vi "7-CleanFP2ndMode.vi"   [LabVIEW 2015, in "TestVIs.lvlib"]
uses:
  TestVIs.lvlib
  <vilib>/Utility/miscctls.llb/LVRectTypeDef.ctl
  <vilib>/Utility/traverseref.llb/TRef TravTarget.ctl
  <vilib>/Utility/VariantDataType/Type.ctl
  <vilib>/Utility/VariantDataType/VariantType.lvlib
types:
  T1 = enum32{"Top Edges", "Vertical Centers", "Bottom Edges", "Left Edges", "Horizontal Centers", "Right Edges"}
  T2 = enum32{"Top Edges", "Vertical Centers", "Bottom Edges", "Vertical Gap", "Vertical Compress", "Left Edges", "Horizontal Centers", "Right Edges", "Horizontal Gap", "Horizontal Compress"}
  T3 = typedef "TRef TravTarget.ctl" = enum16{"FP", "BD", "Other"}
  T4 = typedef "LVRectTypeDef.ctl" = cluster{"Left":i16, "Top":i16, "Right":i16, "Bottom":i16}
  T5 = enum16{"Invalid Wire Rule", "Required", "Recommended", "Optional", "Dynamic Dispatch"}
  T6 = enum16{"Invalid Wire Rule", "Required", "Recommended", "Optional", "Dynamic Dispatch"}[]
  T7 = typedef "VariantType.lvlib/Type.ctl" = enum8{"Invalid Type", "Void", "I8", "I16", "I32", "I64", "U8", "U16", "U32", "U64", "Single Float", "Double Float", "Extended Float", "Single Complex", "Double Complex", "Extended Complex", "Enum U8", "Enum U16", "Enum U32", "Enum U64", "Single Float With Unit", "Double Float With Unit", "Extended Float With Unit", "Single Complex with Unit", "Double Complex with Unit", "Extended Complex with Unit", "Boolean", "String", "Path", "Picture", "Tag", "Array", "Cluster", "Variant", "LV Variant", "Waveform", "Timestamp", "Digital Waveform", "Digital Data", "ExpressData", "Refnum", "External Data", "VI", "Poly VI", "LabVIEW Class Instance", "Fixed Point"}
  T8 = cluster{refnum<vi>, "MasterRect":T4, "Type Enum":T7}
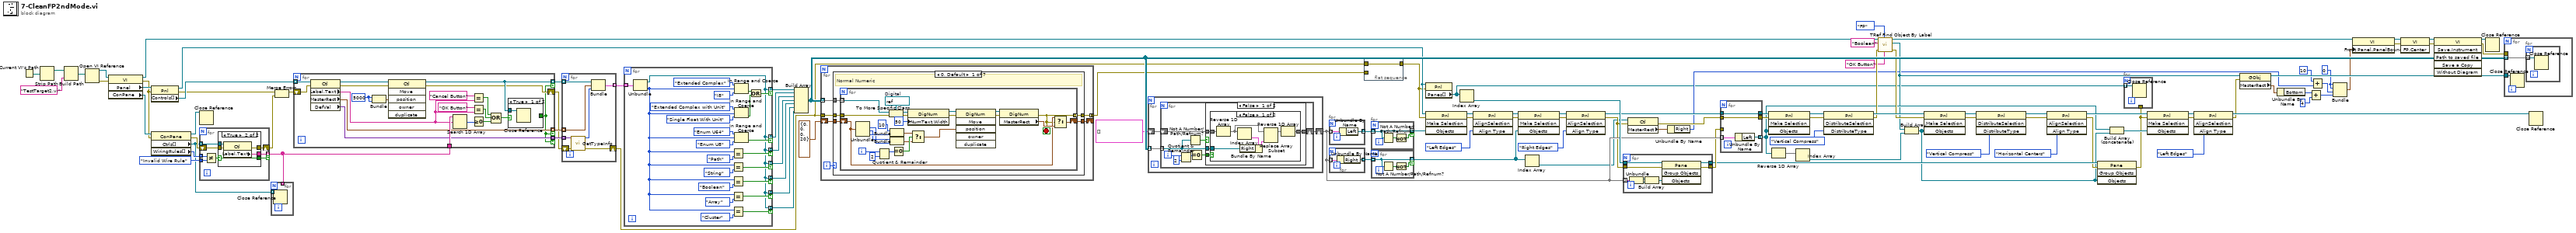
[diagram p0: block diagram]
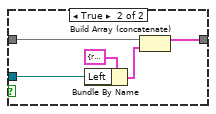
[diagram p2: hidden frame]
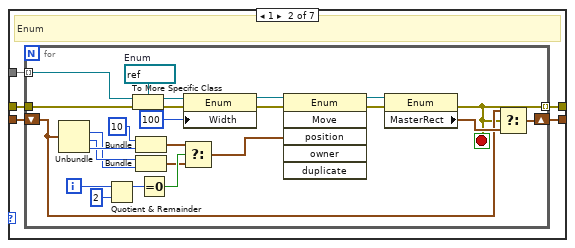
[diagram p4: hidden frame]
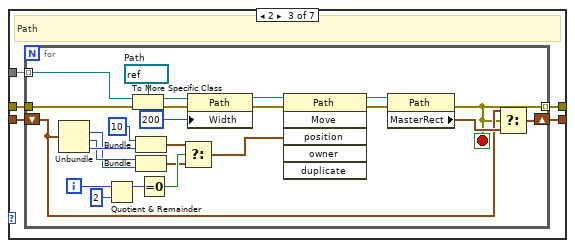
[diagram p5: hidden frame]
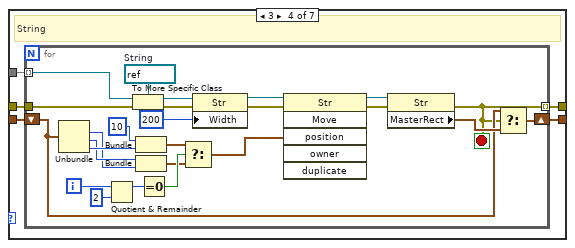
[diagram p6: hidden frame]
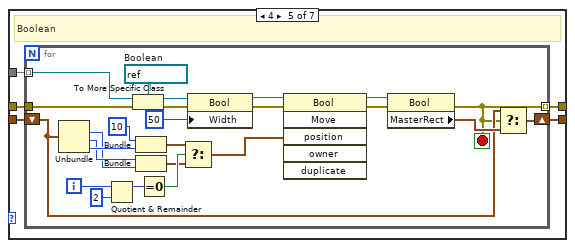
[diagram p7: hidden frame]
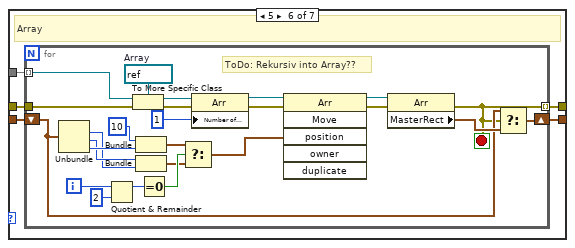
[diagram p8: hidden frame]
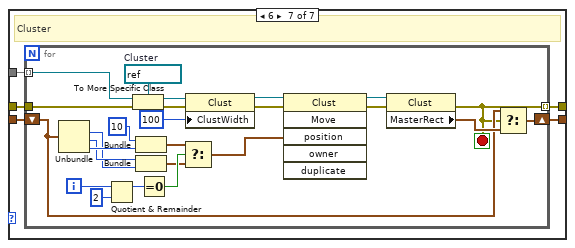
[diagram p9: hidden frame]
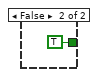
[diagram p10: hidden frame]
diagram:
  w19 = i16 0 ("y")
  n1 = Current VI's Path() -> (path=w106:path)
  n2 = Strip Path(path=w106) -> (stripped path=w109:path)  [unwired: 1 out]
  n3 = Build Path(base path=w109, name or relative path="TestTarget2.vi") -> (appended path=w107:path)
  n4 = Open VI Reference(vi path=w107) -> (vi reference=w93:refnum<vi>, error out=w92:errorcluster)  [unwired: 5 in]
  n5 = property class="VI"(reference=w93, error in=w92) -> (reference out=w52:refnum<vi>, error out=w103:errorcluster, "Panel"=w105:refnum<vi>, "ConPane"=w104:refnum<vi>)
  n6 = property class="Pnl"(reference=w105, error in=w103) -> (reference out=w64:refnum<vi>, error out=w100:errorcluster, "Controls[]"=w101:refnum<vi>[])
  n7 = property class="ConPane"(reference=w104, error in=w103) -> (reference out=w91:refnum<vi>, error out=w102:errorcluster, "Ctrls[]"=w8:refnum<vi>[], "WiringRules[]"=w89:T6)
  n8 = Close Reference(reference=w91) -> ()  [unwired: 1 in, 1 out]
  n9 = for {
    tunnel: w8 -> [w117] mode=indexing
    shift-right: [w115] -> w98
    shift-left: w102 -> [w116]
    tunnel: [w114] -> w7 mode=indexing if=w110
    tunnel: w89 -> [w112] mode=indexing
    tunnel: T5."Invalid Wire Rule" ("Wire Rule") -> [w111]
    n10 = Not Equal?(x=w112, y=w111) -> (x != y?=w113:bool)
    n11 = case shown="True" w113 {
      selector: w113 -> [w118 w120]
      tunnel: w117 -> [_ w124]
      tunnel: w116 -> [w119 w123]
      tunnel: [w119 w122] -> w115
      tunnel: [_ w121] -> w114
      tunnel: [w118 w120] -> w110
      frame False {
      }
      frame True {
        n12 = property class="Ctl"(reference=w124, error in=w123) -> (error out=w122:errorcluster, "Label.Text"=w121:string)  [unwired: 1 out]
      }
    }
  }
  n13 = for {
    tunnel: w8 -> [w125] mode=indexing
    tunnel: w7 -> [_] mode=indexing
    n14 = Close Reference(reference=w125) -> ()  [unwired: 1 in, 1 out]
  }
  n15 = Merge Errors(w100, w98) -> (w99:errorcluster)
  n16 = for {
    tunnel: w101 -> [w145] mode=indexing
    shift-right: [w137] -> w94
    shift-left: w99 -> [w144]
    tunnel: w7 -> [w143]
    tunnel: [w138] -> w95 mode=indexing if=w134
    tunnel: [w136] -> w96 mode=indexing if=w134
    tunnel: [w135] -> w97 mode=indexing if=w134
    w142 = i16 5000 ("x")
    n17 = property class="Ctl"(reference=w145, error in=w144) -> (reference out=w139:refnum<vi>, error out=w140:errorcluster, "Label.Text"=w132:string, "MasterRect"=w136:T4, "DefVal"=w135:variant)
    n18 = Bundle("x"=w142, "x"=w142) -> (w141:cluster{"x":i16, "x":i16})  [unwired: 1 in]
    n19 = invoke class="Ctl" method="Move"(reference=w139, error in=w140, "position"=w141) -> (reference out=w138:refnum<vi>, error out=w137:errorcluster)  [unwired: 3 in, 4 out]
    n20 = Search 1D Array(1D array=w143, element=w132) -> (index of element=w133:i32)  [unwired: 1 in]
    n21 = Equal?(x="Cancel Button", y=w132) -> (x = y?=w131:bool)
    n22 = Equal?(x="OK Button", y=w132) -> (x = y?=w130:bool)
    n23 = Greater Or Equal To 0?(x=w133) -> (x >= 0?=w129:bool)
    n24 = Compound Arithmetic op=OR(w131, w130, w129) -> (w128:bool)
    n25 = case shown="True" w128 {
      tunnel: w138 -> [w146 _]
      tunnel: [_ TRUE] -> w134
      frame True {
        n26 = Close Reference(reference=w146) -> ()  [unwired: 1 in, 1 out]
      }
      frame False {
      }
    }
  }
  n27 = for {
    tunnel: w97 -> [w154] mode=indexing
    tunnel: w96 -> [w152] mode=indexing
    tunnel: w95 -> [w153] mode=indexing
    tunnel: [w151] -> w90 mode=indexing
    shift-right: [w149] -> w66
    shift-left: w94 -> [w150]
    n28 = call <vilib>:"GetTypeInfo.vi"("error in (no error)"=w150, "Variant"=w154) -> ("error out"=w149:errorcluster, "Type Enum"=w148:T7)  [unwired: 5 in, 3 out]
    n29 = Bundle(w153, "MasterRect"=w152, "Type Enum"=w148) -> (w151:T8)  [unwired: 1 in]
  }
  n30 = for {
    tunnel: w90 -> [w157] mode=indexing
    tunnel: [w155] -> w87 mode=indexing if=w171
    tunnel: [w155] -> w86 mode=indexing if=w168
    tunnel: [w155] -> w85 mode=indexing if=w158
    tunnel: [w155] -> w82 mode=indexing if=w166
    tunnel: [w155] -> w81 mode=indexing if=w163
    tunnel: [w155] -> w80 mode=indexing if=w162
    tunnel: [w155] -> w83 mode=indexing if=w156
    n31 = Unbundle(w157) -> (w155:refnum<vi>, "Type Enum"=w159:T7)  [unwired: 1 out]
    n32 = Equal?(x=w159, y=Type."Path" ("Type Enum")) -> (x = y?=w158:bool)
    n33 = Equal?(x=w159, y=Type."String" ("Type Enum")) -> (x = y?=w156:bool)
    n34 = Equal?(x=w159, y=Type."Boolean" ("Type Enum")) -> (x = y?=w166:bool)
    n35 = Equal?(x=w159, y=Type."Array" ("Type Enum")) -> (x = y?=w163:bool)
    n36 = Equal?(x=w159, y=Type."Cluster" ("Type Enum")) -> (x = y?=w162:bool)
    n37 = In Range and Coerce(upper limit=Type."Extended Complex" ("Type Enum"), x=w159, lower limit=Type."I8" ("Type Enum")) -> (In Range?=w173:bool)  [unwired: 1 out]
    n38 = In Range and Coerce(upper limit=Type."Extended Complex with Unit" ("Type Enum"), x=w159, lower limit=Type."Single Float With Unit" ("Type Enum")) -> (In Range?=w172:bool)  [unwired: 1 out]
    n39 = In Range and Coerce(upper limit=Type."Enum U64" ("Type Enum"), x=w159, lower limit=Type."Enum U8" ("Type Enum")) -> (In Range?=w168:bool)  [unwired: 1 out]
    n40 = Or(x=w173, y=w172) -> (x .or. y?=w171:bool)
  }
  n41 = Build Array(w87, w86, w85, w83, w82, w81, w80) -> (w79:refnum<vi>[][])
  n42 = for {
    tunnel: w79 -> [w182] mode=indexing
    shift-right: [w179] -> _
    shift-left: T4 {"Left"=0, "Top"=0, "Right"=0, "Bottom"=20} ("MasterRect") -> [w180]
    tunnel: w66 -> [w183]
    tunnel: [w178] -> w65 mode=concatenating
    i -> [w181]
    n43 = case shown="0, Default" w181 {
      tunnel: w182 -> [w188 w218 w248 w278 w308 w338 w368]
      tunnel: [w187 w217 w247 w277 w307 w337 w367] -> w178
      tunnel: [w186 w216 w246 w276 w306 w336 w366] -> w179
      tunnel: w183 -> [w185 w215 w245 w275 w305 w335 w365]
      tunnel: w180 -> [w184 w214 w244 w274 w304 w334 w364]
      frame 0, Default {
        # "Normal Numeric"
        n44 = for {
          tunnel: w188 -> [w193] mode=indexing
          shift-right: [w192] -> w186
          shift-left: w184 -> [w190]
          tunnel: w185 -> [w212]
          tunnel: [w189] -> w187 mode=indexing
          i -> [w213]
          stop <- w189 stop-if-true
          w194 = refnum<vi> refnum  # Digital
          n45 = Unbundle(w190) -> ("Top"=w195:i16, "Right"=w196:i16, "Bottom"=w197:i16)  [unwired: 1 out]
          n46 = Quotient & Remainder(x=w213, y=2) -> (x-y*floor(x/y)=w203:i32)  [unwired: 1 out]
          n47 = To More Specific Class(target class=w194, reference=w193, error in=w212) -> (specific class reference=w210:refnum<vi>, error out=w209:errorcluster)
          n48 = Bundle("Top"=i16 10, "Bottom"=w197) -> (w200:cluster{"Top":i16, "Bottom":i16})  [unwired: 1 in]
          n49 = Bundle("Right"=w196, "Top"=w195) -> (w199:cluster{"Right":i16, "Top":i16})  [unwired: 1 in]
          n50 = Equal To 0?(x=w203) -> (x = 0?=w202:bool)
          n51 = property class="DigNum"(reference=w210, error in=w209, "NumText.Width"=u32 50 ("Numeric Text.Size:Width")) -> (reference out=w208:refnum<vi>, error out=w207:errorcluster)
          n52 = Select(t=w200, s=w202, f=w199) -> (s? t:f=w201:cluster{"Right":i16, "Top":i16})
          n53 = invoke class="DigNum" method="Move"(reference=w208, error in=w207, "position"=w201) -> (reference out=w205:refnum<vi>, error out=w204:errorcluster)  [unwired: 3 in, 4 out]
          n54 = property class="DigNum"(reference=w205, error in=w204) -> (error out=w189:errorcluster, "MasterRect"=w191:T4)  [unwired: 1 out]
          n55 = Select(t=w190, s=w189, f=w191) -> (s? t:f=w192:T4)
        }
      }
      frame 1 {
        # "Enum"
        n56 = for {
          tunnel: w218 -> [w223] mode=indexing
          shift-right: [w222] -> w216
          shift-left: w214 -> [w220]
          tunnel: w215 -> [w242]
          tunnel: [w219] -> w217 mode=indexing
          i -> [w243]
          stop <- w219 stop-if-true
          w224 = refnum<vi> refnum  # Enum
          n57 = Unbundle(w220) -> ("Top"=w225:i16, "Right"=w226:i16, "Bottom"=w227:i16)  [unwired: 1 out]
          n58 = Quotient & Remainder(x=w243, y=2) -> (x-y*floor(x/y)=w233:i32)  [unwired: 1 out]
          n59 = To More Specific Class(target class=w224, reference=w223, error in=w242) -> (specific class reference=w240:refnum<vi>, error out=w239:errorcluster)
          n60 = Bundle("Top"=i16 10, "Bottom"=w227) -> (w230:cluster{"Top":i16, "Bottom":i16})  [unwired: 1 in]
          n61 = Bundle("Right"=w226, "Top"=w225) -> (w229:cluster{"Right":i16, "Top":i16})  [unwired: 1 in]
          n62 = Equal To 0?(x=w233) -> (x = 0?=w232:bool)
          n63 = Select(t=w230, s=w232, f=w229) -> (s? t:f=w231:cluster{"Right":i16, "Top":i16})
          n64 = property class="Enum"(reference=w240, error in=w239, "Width"=u32 100 ("Numeric Text.Size:Width")) -> (reference out=w238:refnum<vi>, error out=w237:errorcluster)
          n65 = invoke class="Enum" method="Move"(reference=w238, error in=w237, "position"=w231) -> (reference out=w235:refnum<vi>, error out=w234:errorcluster)  [unwired: 3 in, 4 out]
          n66 = property class="Enum"(reference=w235, error in=w234) -> (error out=w219:errorcluster, "MasterRect"=w221:T4)  [unwired: 1 out]
          n67 = Select(t=w220, s=w219, f=w221) -> (s? t:f=w222:T4)
        }
      }
      frame 2 {
        # "Path"
        n68 = for {
          tunnel: w248 -> [w253] mode=indexing
          shift-right: [w252] -> w246
          shift-left: w244 -> [w250]
          tunnel: w245 -> [w272]
          tunnel: [w249] -> w247 mode=indexing
          i -> [w273]
          stop <- w249 stop-if-true
          w254 = refnum<vi> refnum  # Path
          n69 = Unbundle(w250) -> ("Top"=w255:i16, "Right"=w256:i16, "Bottom"=w257:i16)  [unwired: 1 out]
          n70 = Quotient & Remainder(x=w273, y=2) -> (x-y*floor(x/y)=w263:i32)  [unwired: 1 out]
          n71 = To More Specific Class(target class=w254, reference=w253, error in=w272) -> (specific class reference=w270:refnum<vi>, error out=w269:errorcluster)
          n72 = Bundle("Top"=i16 10, "Bottom"=w257) -> (w260:cluster{"Top":i16, "Bottom":i16})  [unwired: 1 in]
          n73 = Bundle("Right"=w256, "Top"=w255) -> (w259:cluster{"Right":i16, "Top":i16})  [unwired: 1 in]
          n74 = Equal To 0?(x=w263) -> (x = 0?=w262:bool)
          n75 = Select(t=w260, s=w262, f=w259) -> (s? t:f=w261:cluster{"Right":i16, "Top":i16})
          n76 = property class="Path"(reference=w270, error in=w269, "Width"=u32 200 ("Numeric Text.Size:Width")) -> (reference out=w268:refnum<vi>, error out=w267:errorcluster)
          n77 = invoke class="Path" method="Move"(reference=w268, error in=w267, "position"=w261) -> (reference out=w265:refnum<vi>, error out=w264:errorcluster)  [unwired: 3 in, 4 out]
          n78 = property class="Path"(reference=w265, error in=w264) -> (error out=w249:errorcluster, "MasterRect"=w251:T4)  [unwired: 1 out]
          n79 = Select(t=w250, s=w249, f=w251) -> (s? t:f=w252:T4)
        }
      }
      frame 3 {
        # "String"
        n80 = for {
          tunnel: w278 -> [w283] mode=indexing
          shift-right: [w282] -> w276
          shift-left: w274 -> [w280]
          tunnel: w275 -> [w302]
          tunnel: [w279] -> w277 mode=indexing
          i -> [w303]
          stop <- w279 stop-if-true
          w284 = refnum<vi> refnum  # String
          n81 = Unbundle(w280) -> ("Top"=w285:i16, "Right"=w286:i16, "Bottom"=w287:i16)  [unwired: 1 out]
          n82 = Quotient & Remainder(x=w303, y=2) -> (x-y*floor(x/y)=w293:i32)  [unwired: 1 out]
          n83 = To More Specific Class(target class=w284, reference=w283, error in=w302) -> (specific class reference=w300:refnum<vi>, error out=w299:errorcluster)
          n84 = Bundle("Top"=i16 10, "Bottom"=w287) -> (w290:cluster{"Top":i16, "Bottom":i16})  [unwired: 1 in]
          n85 = Bundle("Right"=w286, "Top"=w285) -> (w289:cluster{"Right":i16, "Top":i16})  [unwired: 1 in]
          n86 = Equal To 0?(x=w293) -> (x = 0?=w292:bool)
          n87 = Select(t=w290, s=w292, f=w289) -> (s? t:f=w291:cluster{"Right":i16, "Top":i16})
          n88 = property class="Str"(reference=w300, error in=w299, "Width"=u32 200 ("Numeric Text.Size:Width")) -> (reference out=w298:refnum<vi>, error out=w297:errorcluster)
          n89 = invoke class="Str" method="Move"(reference=w298, error in=w297, "position"=w291) -> (reference out=w295:refnum<vi>, error out=w294:errorcluster)  [unwired: 3 in, 4 out]
          n90 = property class="Str"(reference=w295, error in=w294) -> (error out=w279:errorcluster, "MasterRect"=w281:T4)  [unwired: 1 out]
          n91 = Select(t=w280, s=w279, f=w281) -> (s? t:f=w282:T4)
        }
      }
      frame 4 {
        # "Boolean"
        n92 = for {
          tunnel: w308 -> [w313] mode=indexing
          shift-right: [w312] -> w306
          shift-left: w304 -> [w310]
          tunnel: w305 -> [w332]
          tunnel: [w309] -> w307 mode=indexing
          i -> [w333]
          stop <- w309 stop-if-true
          w314 = refnum<vi> refnum  # Boolean
          n93 = Unbundle(w310) -> ("Top"=w315:i16, "Right"=w316:i16, "Bottom"=w317:i16)  [unwired: 1 out]
          n94 = Quotient & Remainder(x=w333, y=2) -> (x-y*floor(x/y)=w323:i32)  [unwired: 1 out]
          n95 = To More Specific Class(target class=w314, reference=w313, error in=w332) -> (specific class reference=w330:refnum<vi>, error out=w329:errorcluster)
          n96 = Bundle("Top"=i16 10, "Bottom"=w317) -> (w320:cluster{"Top":i16, "Bottom":i16})  [unwired: 1 in]
          n97 = Bundle("Right"=w316, "Top"=w315) -> (w319:cluster{"Right":i16, "Top":i16})  [unwired: 1 in]
          n98 = Equal To 0?(x=w323) -> (x = 0?=w322:bool)
          n99 = Select(t=w320, s=w322, f=w319) -> (s? t:f=w321:cluster{"Right":i16, "Top":i16})
          n100 = property class="Bool"(reference=w330, error in=w329, "Width"=u32 50 ("Numeric Text.Size:Width")) -> (reference out=w328:refnum<vi>, error out=w327:errorcluster)
          n101 = invoke class="Bool" method="Move"(reference=w328, error in=w327, "position"=w321) -> (reference out=w325:refnum<vi>, error out=w324:errorcluster)  [unwired: 3 in, 4 out]
          n102 = property class="Bool"(reference=w325, error in=w324) -> (error out=w309:errorcluster, "MasterRect"=w311:T4)  [unwired: 1 out]
          n103 = Select(t=w310, s=w309, f=w311) -> (s? t:f=w312:T4)
        }
      }
      frame 5 {
        # "Array"
        n104 = for {
          tunnel: w338 -> [w343] mode=indexing
          shift-right: [w342] -> w336
          shift-left: w334 -> [w340]
          tunnel: w335 -> [w362]
          tunnel: [w339] -> w337 mode=indexing
          i -> [w363]
          stop <- w339 stop-if-true
          w344 = refnum<vi> refnum  # Array
          # "ToDo: Rekursiv into Array??"
          n105 = Unbundle(w340) -> ("Top"=w345:i16, "Right"=w346:i16, "Bottom"=w347:i16)  [unwired: 1 out]
          n106 = Quotient & Remainder(x=w363, y=2) -> (x-y*floor(x/y)=w353:i32)  [unwired: 1 out]
          n107 = To More Specific Class(target class=w344, reference=w343, error in=w362) -> (specific class reference=w360:refnum<vi>, error out=w359:errorcluster)
          n108 = Bundle("Top"=i16 10, "Bottom"=w347) -> (w350:cluster{"Top":i16, "Bottom":i16})  [unwired: 1 in]
          n109 = Bundle("Right"=w346, "Top"=w345) -> (w349:cluster{"Right":i16, "Top":i16})  [unwired: 1 in]
          n110 = Equal To 0?(x=w353) -> (x = 0?=w352:bool)
          n111 = Select(t=w350, s=w352, f=w349) -> (s? t:f=w351:cluster{"Right":i16, "Top":i16})
          n112 = property class="Arr"(reference=w360, error in=w359, "Number of Columns"=u32 1 ("Numeric Text.Size:Width")) -> (reference out=w358:refnum<vi>, error out=w357:errorcluster)
          n113 = invoke class="Arr" method="Move"(reference=w358, error in=w357, "position"=w351) -> (reference out=w355:refnum<vi>, error out=w354:errorcluster)  [unwired: 3 in, 4 out]
          n114 = property class="Arr"(reference=w355, error in=w354) -> (error out=w339:errorcluster, "MasterRect"=w341:T4)  [unwired: 1 out]
          n115 = Select(t=w340, s=w339, f=w341) -> (s? t:f=w342:T4)
        }
      }
      frame 6 {
        # "Cluster"
        n116 = for {
          tunnel: w368 -> [w373] mode=indexing
          shift-right: [w372] -> w366
          shift-left: w364 -> [w370]
          tunnel: w365 -> [w392]
          tunnel: [w369] -> w367 mode=indexing
          i -> [w393]
          stop <- w369 stop-if-true
          w374 = refnum<vi> refnum  # Cluster
          n117 = Unbundle(w370) -> ("Top"=w375:i16, "Right"=w376:i16, "Bottom"=w377:i16)  [unwired: 1 out]
          n118 = Quotient & Remainder(x=w393, y=2) -> (x-y*floor(x/y)=w383:i32)  [unwired: 1 out]
          n119 = To More Specific Class(target class=w374, reference=w373, error in=w392) -> (specific class reference=w390:refnum<vi>, error out=w389:errorcluster)
          n120 = Bundle("Top"=i16 10, "Bottom"=w377) -> (w380:cluster{"Top":i16, "Bottom":i16})  [unwired: 1 in]
          n121 = Bundle("Right"=w376, "Top"=w375) -> (w379:cluster{"Right":i16, "Top":i16})  [unwired: 1 in]
          n122 = Equal To 0?(x=w383) -> (x = 0?=w382:bool)
          n123 = Select(t=w380, s=w382, f=w379) -> (s? t:f=w381:cluster{"Right":i16, "Top":i16})
          n124 = property class="Clust"(reference=w390, error in=w389, "ClustWidth"=u32 100 ("Numeric Text.Size:Width")) -> (reference out=w388:refnum<vi>, error out=w387:errorcluster)
          n125 = invoke class="Clust" method="Move"(reference=w388, error in=w387, "position"=w381) -> (reference out=w385:refnum<vi>, error out=w384:errorcluster)  [unwired: 3 in, 4 out]
          n126 = property class="Clust"(reference=w385, error in=w384) -> (error out=w369:errorcluster, "MasterRect"=w371:T4)  [unwired: 1 out]
          n127 = Select(t=w370, s=w369, f=w371) -> (s? t:f=w372:T4)
        }
      }
    }
  }
  n128 = for {
    tunnel: w79 -> [w396] mode=indexing
    shift-right: [w394] -> w61
    shift-left: cluster{"Left":refnum<vi>, "Right":refnum<vi>}[] [] -> [w395]
    n129 = for {
      tunnel: w396 -> [w398] mode=indexing
      shift-right: [w399] -> w394
      shift-left: w395 -> [w400]
      i -> [w402]
      n130 = Quotient & Remainder(x=w402, y=2) -> (x-y*floor(x/y)=w403:i32)  [unwired: 1 out]
      n131 = Not A Number/Path/Refnum?(number/path/refnum=w398) -> (NaN/Path/Refnum?=w397:bool)
      n132 = Equal To 0?(x=w403) -> (x = 0?=w401:bool)
      n133 = case shown="False" w397 {
        tunnel: w401 -> [w408 _]
        tunnel: w400 -> [w407 w421]
        tunnel: [w406 w421] -> w399
        tunnel: w398 -> [w405 _]
        frame False {
          n134 = case shown="False" w408 {
            tunnel: w407 -> [w415 w420]
            tunnel: [w412 w419] -> w406
            tunnel: w405 -> [w409 w418]
            frame False {
              n135 = Reverse 1D Array(array=w415) -> (reversed array=w414:cluster{"Left":refnum<vi>, "Right":refnum<vi>}[])
              n136 = Index Array(array=w414) -> (element=w411:cluster{"Left":refnum<vi>, "Right":refnum<vi>})  [unwired: 1 in]
              n137 = Bundle By Name(cluster=w411, "Right"=w409) -> (w410:cluster{"Left":refnum<vi>, "Right":refnum<vi>})
              n138 = Replace Array Subset(array=w414, new element=w410) -> (w413:cluster{"Left":refnum<vi>, "Right":refnum<vi>}[])  [unwired: 1 in]
              n139 = Reverse 1D Array(array=w413) -> (reversed array=w412:cluster{"Left":refnum<vi>, "Right":refnum<vi>}[])
            }
            frame True {
              n140 = Bundle By Name(cluster=cluster{"Left":refnum<vi>, "Right":refnum<vi>} {"Left"=refnum, "Right"=refnum}, "Left"=w418) -> (w416:cluster{"Left":refnum<vi>, "Right":refnum<vi>})
              n141 = Build Array (concatenate)(w420, w416) -> (w419:cluster{"Left":refnum<vi>, "Right":refnum<vi>}[])
            }
          }
        }
        frame True {
        }
      }
    }
  }
  n142 = for {
    tunnel: w61 -> [w423] mode=indexing
    tunnel: [w422] -> w68 mode=indexing
    n143 = Unbundle By Name(w423) -> ("Left"=w422:refnum<vi>)
  }
  n144 = for {
    tunnel: w61 -> [w425] mode=indexing
    tunnel: [w424] -> w69 mode=indexing
    n145 = Unbundle By Name(w425) -> ("Right"=w424:refnum<vi>)
  }
  n146 = flat-sequence {
    tunnel: w66 -> [w426]
    tunnel: [w426] -> w63
    tunnel: w65 -> [_]
    frame #0 {
    }
  }
  n147 = for {
    tunnel: w68 -> [w427] mode=indexing
    tunnel: [w427] -> w67 mode=indexing if=w428
    n148 = Not A Number/Path/Refnum?(number/path/refnum=w427) -> (NaN/Path/Refnum?=w429:bool)
    n149 = Not(x=w429) -> (.not. x?=w428:bool)
  }
  n150 = for {
    tunnel: w69 -> [w430] mode=indexing
    tunnel: [w430] -> w16 mode=indexing if=w431
    n151 = Not A Number/Path/Refnum?(number/path/refnum=w430) -> (NaN/Path/Refnum?=w432:bool)
    n152 = Not(x=w432) -> (.not. x?=w431:bool)
  }
  n153 = property class="Pnl"(reference=w64, error in=w63) -> ("Panes[]"=w5:refnum<vi>[])  [unwired: 2 out]
  n154 = invoke class="Pnl" method="Make Selection"(reference=w64, error in=w63, "Objects"=w67) -> (reference out=w77:refnum<vi>, error out=w76:errorcluster)  [unwired: 1 in, 2 out]
  n155 = Index Array(array=w5) -> (element=w62:refnum<vi>)  [unwired: 1 in]
  n156 = invoke class="Pnl" method="AlignSelection"(reference=w77, error in=w76, "Align Type"=T1."Left Edges") -> (reference out=w71:refnum<vi>, error out=w70:errorcluster)  [unwired: 1 in, 2 out]
  n157 = invoke class="Pnl" method="Make Selection"(reference=w71, error in=w70, "Objects"=w16) -> (reference out=w74:refnum<vi>, error out=w73:errorcluster)  [unwired: 1 in, 2 out]
  n158 = Index Array(array=w16) -> (element=w15:refnum<vi>)  [unwired: 1 in]
  n159 = invoke class="Pnl" method="AlignSelection"(reference=w74, error in=w73, "Align Type"=T1."Right Edges") -> (reference out=w60:refnum<vi>, error out=w18:errorcluster)  [unwired: 1 in, 2 out]
  n160 = for {
    tunnel: w61 -> [w439] mode=indexing
    tunnel: w62 -> [w440]
    tunnel: w18 -> [w435]
    tunnel: [w434] -> w54
    tunnel: [w433] -> w38
    n161 = Unbundle(w439) -> ("Left"=w438:refnum<vi>, "Right"=w437:refnum<vi>)
    n162 = Build Array(w438, w437) -> (w436:refnum<vi>[])
    n163 = invoke class="Pane" method="Group Objects"(reference=w440, error in=w435, "Objects"=w436) -> (reference out=w433:refnum<vi>, error out=w434:errorcluster)  [unwired: 1 in, 2 out]
  }
  n164 = property class="Ctl"(reference=w15, error in=w18) -> (error out=w17:errorcluster, "MasterRect"=w14:T4)  [unwired: 1 out]
  n165 = Unbundle By Name(w14) -> ("Right"=w11:i16)
  n166 = for {
    tunnel: w61 -> [w444] mode=indexing
    tunnel: w60 -> [w443]
    tunnel: [w443] -> w59
    tunnel: w17 -> [w441]
    tunnel: [w442] -> w29 mode=indexing
    tunnel: [w441] -> w58
    tunnel: w54 -> [_]
    n167 = Unbundle By Name(w444) -> ("Left"=w442:refnum<vi>)
  }
  n168 = invoke class="Pnl" method="Make Selection"(reference=w59, error in=w58, "Objects"=w29) -> (reference out=w57:refnum<vi>, error out=w56:errorcluster)  [unwired: 1 in, 2 out]
  n169 = Reverse 1D Array(array=w29) -> (reversed array=w44:refnum<vi>[])
  n170 = Index Array(array=w44) -> (element=w43:refnum<vi>)  [unwired: 1 in]
  n171 = invoke class="Pnl" method="DistributeSelection"(reference=w57, error in=w56, "DistributeType"=T2."Vertical Compress") -> (reference out=w53:refnum<vi>, error out=w51:errorcluster)  [unwired: 1 in, 2 out]
  n172 = call <vilib>:"TRef Find Object By Label.vi"("Label"="OK Button", "Traverse Target"=TRef_TravTarget."FP", "error in (no error)"=w51, "Class Name"="Boolean", "VI Ref"=w52) -> ("error out"=w39:errorcluster, "Found Obj Ref"=w27:refnum<vi>, "dup VI Ref"=w28:refnum<vi>)  [unwired: 3 in, 1 out]
  n173 = Build Array(w27, w43) -> (w31:refnum<vi>[])
  n174 = invoke class="Pnl" method="Make Selection"(reference=w53, error in=w39, "Objects"=w31) -> (reference out=w47:refnum<vi>, error out=w46:errorcluster)  [unwired: 1 in, 2 out]
  n175 = invoke class="Pnl" method="DistributeSelection"(reference=w47, error in=w46, "DistributeType"=T2."Vertical Compress") -> (reference out=w42:refnum<vi>, error out=w41:errorcluster)  [unwired: 1 in, 2 out]
  n176 = invoke class="Pnl" method="AlignSelection"(reference=w42, error in=w41, "Align Type"=T1."Horizontal Centers") -> (reference out=w34:refnum<vi>, error out=w37:errorcluster)  [unwired: 1 in, 2 out]
  n177 = invoke class="Pane" method="Group Objects"(reference=w38, error in=w37, "Objects"=w31) -> (error out=w6:errorcluster)  [unwired: 1 in, 3 out]
  n178 = Build Array (concatenate)(w29, w31) -> (w30:refnum<vi>[])
  n179 = for {
    tunnel: w6 -> [_]
    tunnel: w5 -> [w445] mode=indexing
    n180 = Close Reference(reference=w445) -> ()  [unwired: 1 in, 1 out]
  }
  n181 = invoke class="Pnl" method="Make Selection"(reference=w34, error in=w6, "Objects"=w30) -> (reference out=w36:refnum<vi>, error out=w35:errorcluster)  [unwired: 1 in, 2 out]
  n182 = invoke class="Pnl" method="AlignSelection"(reference=w36, error in=w35, "Align Type"=T1."Left Edges") -> (reference out=w33:refnum<vi>, error out=w25:errorcluster)  [unwired: 1 in, 2 out]
  n183 = property class="GObj"(reference=w27, error in=w25) -> (reference out=w26:refnum<vi>, "MasterRect"=w24:T4)  [unwired: 1 out]
  n184 = Unbundle By Name(w24) -> ("Bottom"=w23:i16)
  n185 = Add(x=w23, y=i16 4) -> (x+y=w20:i16)
  n186 = Add(x=i16 10 ("y"), y=w11) -> (x+y=w13:i16)
  n187 = Bundle("y"=w19, "y"=w19, w13, w20) -> (w21:cluster{"y":i16, "y":i16, i16, i16})  [unwired: 1 in]
  n188 = property class="VI"(reference=w28, "Front Panel.PanelBounds"=w21) -> (reference out=w10:refnum<vi>, error out=w9:errorcluster)  [unwired: 1 in]
  n189 = invoke class="VI" method="FP.Center"(reference=w10, error in=w9) -> (reference out=w4:refnum<vi>, error out=w2:errorcluster)  [unwired: 1 in, 1 out]
  n190 = invoke class="VI" method="Save.Instrument"(reference=w4, error in=w2) -> (reference out=w3:refnum<vi>, error out=w1:errorcluster)  [unwired: 4 in, 4 out]
  n191 = Close Reference(reference=w3) -> ()  [unwired: 1 in, 1 out]
  n192 = for {
    tunnel: w79 -> [w447] mode=indexing
    tunnel: w1 -> [_]
    tunnel: w26 -> [w446]
    n193 = Close Reference(reference=w446) -> ()  [unwired: 1 in, 1 out]
    n194 = for {
      tunnel: w447 -> [w448] mode=indexing
      n195 = Close Reference(reference=w448) -> ()  [unwired: 1 in, 1 out]
    }
  }
  n196 = Close Reference(reference=w33) -> ()  [unwired: 1 in, 1 out]
